vi "ScanDone.vi"(8 "error in (no error)":errorcluster, 11 "ControllerComm.lvlib:TranslationStageUI.lvclass":refnum<class "TranslationStageUI.lvclass">) -> (0 "error out":errorcluster, 3 "ControllerComm.lvlib:TranslationStageUI.lvclass":refnum<class "TranslationStageUI.lvclass">)   [LabVIEW 2023, in "TranslationStage_UI.lvlib" / "TranslationStageUI.lvclass"]
uses:
  TranslationStageUI.lvclass
  TranslationStageUI.lvclass/TranslationStageUI.ctl
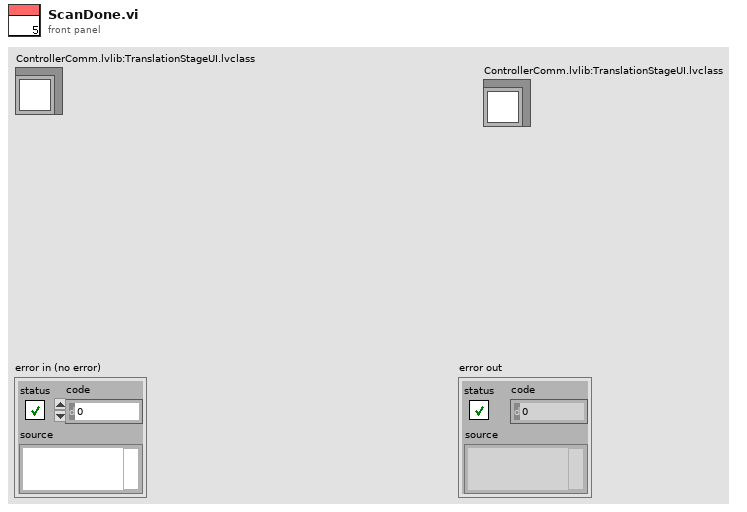
[diagram p1: front panel]
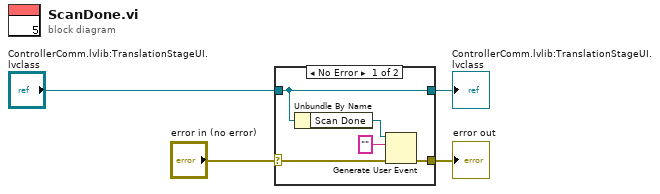
[diagram p0: block diagram]
diagram:
  n1 = case shown="No Error" "error in (no error)" {
    selector: "error in (no error)" -> [w5 w11]
    tunnel: [w6 w11] -> w1
    tunnel: [w9 w10] -> w3
    tunnel: "ControllerComm.lvlib:TranslationStageUI.lvclass" -> [w9 w10]
    frame No Error {
      n2 = Unbundle By Name(w9) -> ("Scan Done"=w8:refnum<user-event>)
      n3 = Generate User Event(user event=w8, event data cluster="" ("event data"), error in=w5) -> (error out=w6:errorcluster)  [unwired: 1 in, 1 out]
    }
    frame Error {
    }
  }
  "error out" <- w1
  "ControllerComm.lvlib:TranslationStageUI.lvclass" <- w3
